vi "Load Test Case Login Credentials.vi"(8 "error in":errorcluster, 10 "Device Model":enum16{"cRIO-9068"}(ring), 11 "Test Case Configuration File Directory":path=path "C:/Github/SMI/source/SMI Tests/User Defined Test VIs/Test Case Configuration Files") -> (0 "error out":errorcluster, 1 "Password":string, 2 "Username":string, 3 "IP Address":string)   [LabVIEW 2015, in "SMI Tests.lvlib"]
uses:
  <vilib>/Utility/config.llb/Read Key (String).vi
  SMI Tests.lvlib
  <vilib>/Utility/config.llb/NI_LVConfig.lvlib
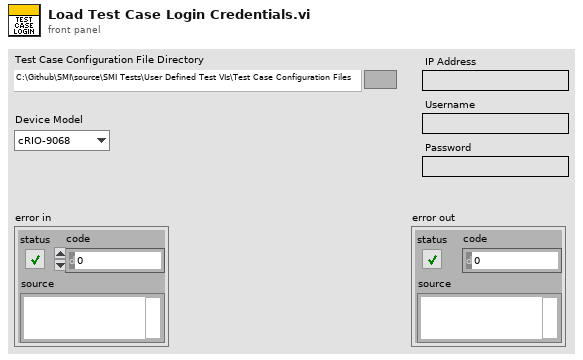
[diagram p1: front panel]
types:
  T1 = typedef "NI_LVConfig.lvlib/Config Data RefNum.ctl" = refnum<k1>
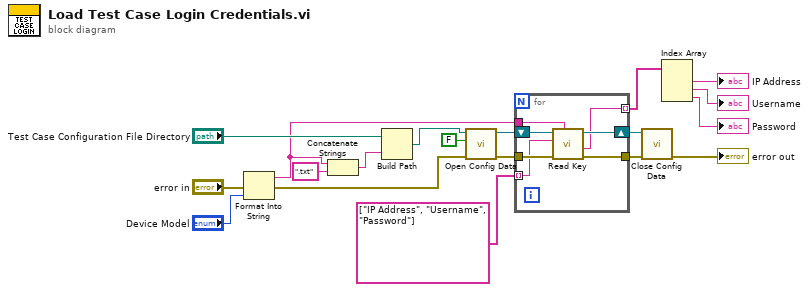
[diagram p0: block diagram]
diagram:
  n1 = Format Into String(error in="error in", "Device Model") -> (resulting string=w2:string, error out=w16:errorcluster)  [unwired: 2 in]
  n2 = Concatenate Strings(w2, ".txt" ("string")) -> (w1:string)
  n3 = Build Path(base path="Test Case Configuration File Directory", name or relative path=w1) -> (appended path=w15:path)
  n4 = call <vilib>:"Open Config Data.vi"("error in (no error)"=w16, "create file if necessary (T)"=FALSE, "configuration file path"=w15) -> ("error out"=w12:errorcluster, "refnum"=w13:T1)  [unwired: 6 in, 1 out]
  n5 = for {
    tunnel: w12 -> [w25]
    tunnel: w2 -> [w24]
    tunnel: string[] ["IP Address", "Username", "Password"] -> [w23] mode=indexing
    shift-right: [w22] -> w8
    shift-left: w13 -> [w26]
    tunnel: [w21] -> w9
    tunnel: [w20] -> w7 mode=indexing
    n6 = call-poly <vilib>:"Read Key.vi"("section"=w24, "error in (no error)"=w25, "key"=w23, "refnum"=w26) -> ("error out"=w21:errorcluster, "value"=w20:string, "refnum out"=w22:T1)  [unwired: 4 in, 1 out]
  }
  n7 = call <vilib>:"Close Config Data.vi"("error in (no error)"=w9, "refnum"=w8) -> ("error out"=→"error out":errorcluster)  [unwired: 8 in, 1 out]
  n8 = Index Array(array=w7) -> (element #1=→"IP Address":string, element #2=→"Username":string, element #3=→"Password":string)  [unwired: 3 in]
